vi "Update Phase Data in MeasDataQ.vi"(6 "UpdateTS (T)":bool=TRUE, 8 "error in (no error)":errorcluster, 9 "TimeStamp":timestamp, 10 "Phase":T2, 11 "Phase Data":T1) -> (0 "error out":errorcluster, 3 "InverterWaveformsQ out":T3)   [LabVIEW 2019]
doc: "Developed by Kevin Thompson\nThompson Engineering, LLC\nkevin@thompsonengineering.net"
uses:
  TD MeasData--cluster.ctl
  TD MeasData QRef.ctl
  GBL DataQ Ref.vi
  DataTypes/InverterData--cluster.ctl
  DataTypes/InverterPhaseData--cluster.ctl
  DataTypes/Phase Selection--enum.ctl
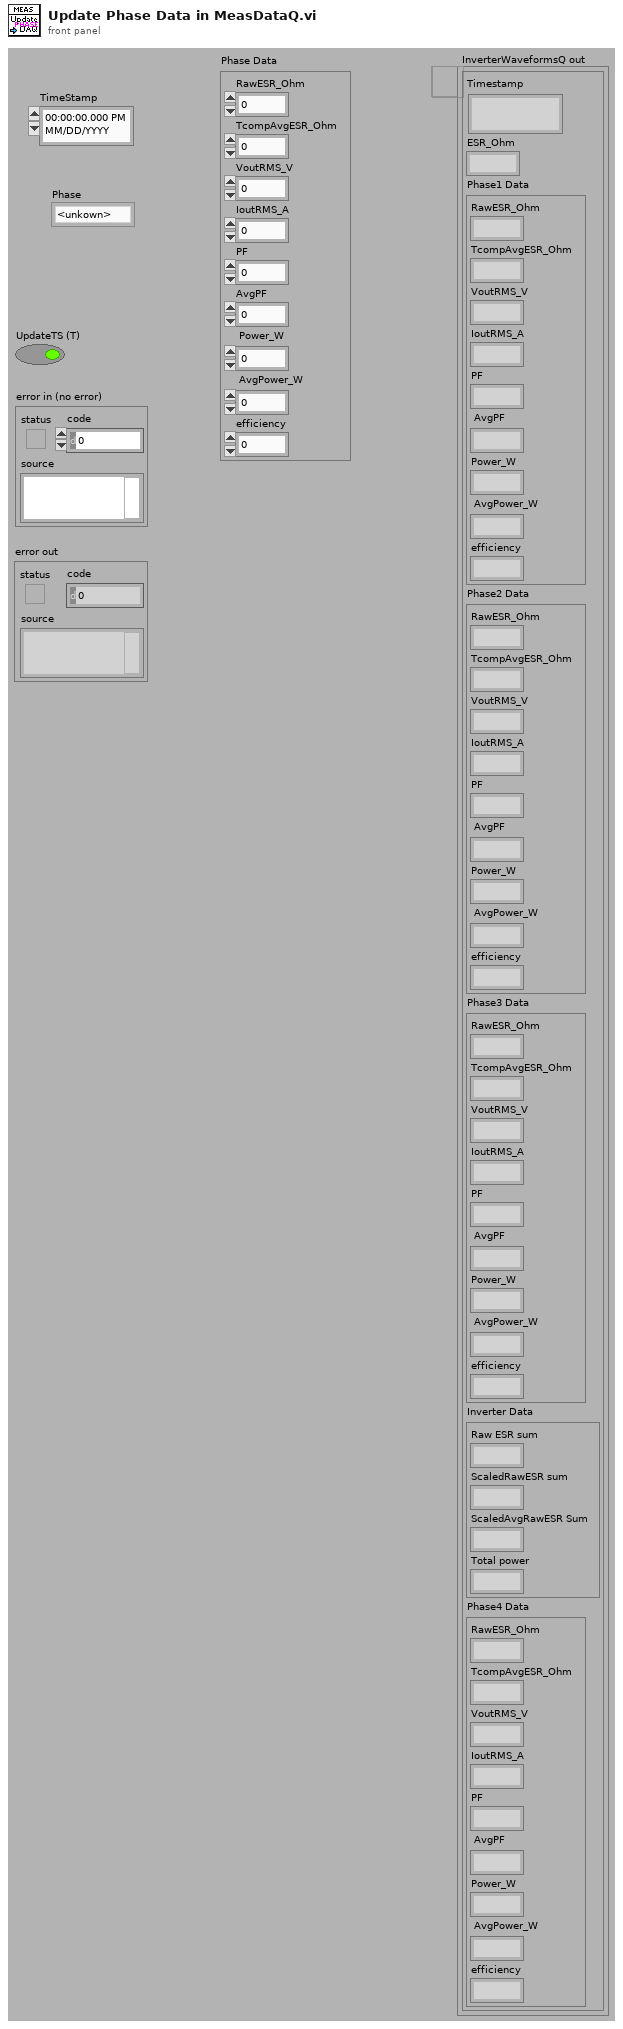
[diagram p1: front panel]
types:
  T1 = typedef "InverterPhaseData--cluster.ctl" = cluster{"RawESR_Ohm":dbl, "TcompAvgESR_Ohm":dbl, "VoutRMS_V":dbl, "IoutRMS_A":dbl, "PF":dbl, "AvgPF":dbl, "Power_W":dbl, "AvgPower_W":dbl, "efficiency":dbl}
  T2 = typedef "Phase Selection--enum.ctl" = enum16{"<unkown>", "Phase 1", "Phase 2", "Phase 3", "Single"}
  T3 = typedef "TD MeasData QRef.ctl" = refnum<queue>
  T4 = typedef "TD MeasData--cluster.ctl" = cluster{"Timestamp":timestamp, "ESR_Ohm":dbl, "Phase1 Data":T1, "Phase2 Data":T1, "Phase3 Data":T1, "Inverter Data":T5, "Phase4 Data":T1}
  T5 = typedef "InverterData--cluster.ctl" = cluster{"Raw ESR sum":dbl, "ScaledRawESR sum":dbl, "ScaledAvgRawESR Sum":dbl, "Total power":dbl}
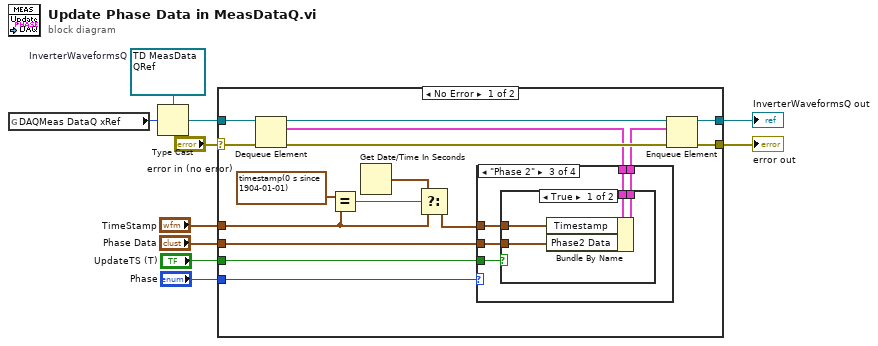
[diagram p0: block diagram]
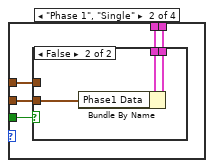
[diagram p3: hidden frame]
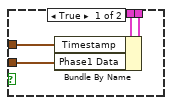
[diagram p4: hidden frame]
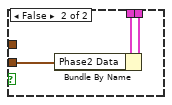
[diagram p5: hidden frame]
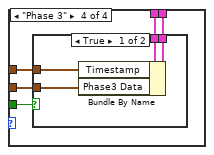
[diagram p6: hidden frame]
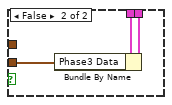
[diagram p7: hidden frame]
diagram:
  w7 = T3 refnum  # InverterWaveformsQ
  n1 = global read "GBL DataQ Ref.vi" "DAQMeas DataQ xRef"() -> (w4:u32)
  n2 = Type Cast(type=w7, x=w4) -> (*(type *) &x=w6:T3)
  n3 = case shown="No Error" "error in (no error)" {
    selector: "error in (no error)" -> [w21 w64]
    tunnel: w6 -> [w26 w65]
    tunnel: [w23 w64] -> w10
    tunnel: [w22 w65] -> w9
    tunnel: "TimeStamp" -> [w16 _]
    tunnel: "Phase Data" -> [w12 _]
    tunnel: "UpdateTS (T)" -> [w13 _]
    tunnel: "Phase" -> [w11 _]
    frame No Error {
      n4 = Dequeue Element(queue=w26, error in (no error)=w21) -> (queue out=w24:T3, element=w20:T4, error out=w25:errorcluster)  [unwired: 1 in, 1 out]
      n5 = Equal?(x=timestamp(0 s since 1904-01-01) ("TimeStamp"), y=w16) -> (x = y?=w17:bool)
      n6 = Get Date/Time In Seconds() -> (seconds since 1Jan1904=w14:timestamp)
      n7 = Select(t=w14, s=w17, f=w16) -> (s? t:f=w15:timestamp)
      n8 = case shown="\"Phase 2\"" w11 {
        tunnel: w20 -> [w27 w32 w44 w56]
        tunnel: [w27 w31 w43 w55] -> w19
        tunnel: w15 -> [_ w30 w42 w54]
        tunnel: w13 -> [_ w29 w41 w53]
        tunnel: w12 -> [_ w28 w40 w52]
        frame Default {
        }
        frame "Phase 1", "Single" {
          n9 = case shown="False" w29 {
            tunnel: w32 -> [w36 w39]
            tunnel: [w35 w38] -> w31
            tunnel: w30 -> [w34 _]
            tunnel: w28 -> [w33 w37]
            frame True {
              n10 = Bundle By Name(cluster=w36, "Timestamp"=w34, "Phase1 Data"=w33) -> (w35:T4)
            }
            frame False {
              n11 = Bundle By Name(cluster=w39, "Phase1 Data"=w37) -> (w38:T4)
            }
          }
        }
        frame "Phase 2" {
          n12 = case shown="True" w41 {
            tunnel: w44 -> [w48 w51]
            tunnel: [w47 w50] -> w43
            tunnel: w42 -> [w46 _]
            tunnel: w40 -> [w45 w49]
            frame True {
              n13 = Bundle By Name(cluster=w48, "Timestamp"=w46, "Phase2 Data"=w45) -> (w47:T4)
            }
            frame False {
              n14 = Bundle By Name(cluster=w51, "Phase2 Data"=w49) -> (w50:T4)
            }
          }
        }
        frame "Phase 3" {
          n15 = case shown="True" w53 {
            tunnel: w56 -> [w60 w63]
            tunnel: [w59 w62] -> w55
            tunnel: w54 -> [w58 _]
            tunnel: w52 -> [w57 w61]
            frame True {
              n16 = Bundle By Name(cluster=w60, "Timestamp"=w58, "Phase3 Data"=w57) -> (w59:T4)
            }
            frame False {
              n17 = Bundle By Name(cluster=w63, "Phase3 Data"=w61) -> (w62:T4)
            }
          }
        }
      }
      n18 = Enqueue Element(queue=w24, element=w19, error in (no error)=w25) -> (queue out=w22:T3, error out=w23:errorcluster)  [unwired: 1 in, 1 out]
    }
    frame Error {
    }
  }
  "InverterWaveformsQ out" <- w9
  "error out" <- w10
